vi "Origin_Input.vi"(4 "error in (no error)":errorcluster, 5 "Measured origin x,y":dbl[](array[numeric])=[0.83, 0.79], 6 "Element In":T4, 7 "Outputmode":u16(ring) items=["Get Path", "Make Layout", "Create TRJs"]) -> (0 "error out":errorcluster, 1 "Init Cluster":T7, 2 "TRJs":T5, 3 "Elements Out":T6(array[cluster]))   [LabVIEW 2009]
panel:
  out "output cluster":T1
  in  "Tab Control":enum32{"Main", "Expert", "Output"}(tab)
  in  "Horizontal Line":T2={"Y-Offset"=-9.0, "Length"=9.0, "X-Offset"=25.5}
  in  "Vertical Line":T3={"X-Offset"=20.0, "Length"=7.0, "Y-Offset"=-8.5}
  in  "stop":bool
  in  "Type":i32=4
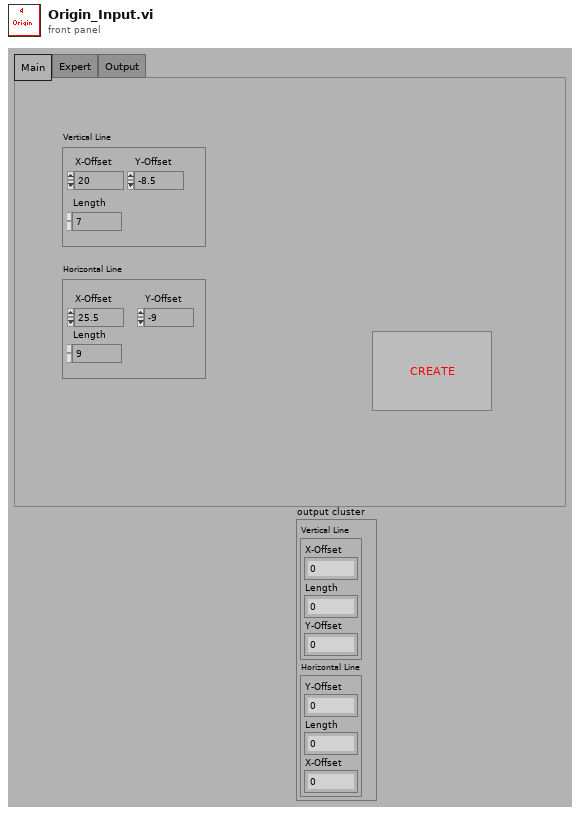
[diagram p1: front panel]
types:
  T1 = cluster{"Vertical Line":cluster{"X-Offset":dbl, "Length":dbl, "Y-Offset":dbl}, "Horizontal Line":cluster{"Y-Offset":dbl, "Length":dbl, "X-Offset":dbl}}
  T2 = cluster{"Y-Offset":dbl, "Length":dbl, "X-Offset":dbl}
  T3 = cluster{"X-Offset":dbl, "Length":dbl, "Y-Offset":dbl}
  T4 = cluster{"Element Name":string, "Type":i32, "Layer per L-Move":i32, "Variant":variant}
  T5 = cluster{"trj file path(1)":path[], "size(s)":i32, dbl[][]}
  T6 = cluster{"Element Name":string, "Type":i32, "Layer per L-Move":i32, "Variant":variant}[]
  T7 = cluster{"path":path, "Button Name":string, "Type":i32}
  T8 = cluster{"Element Name":string, "Value":i32, "Layer per L-Move":i32, "Variant":variant}
  T9 = cluster{"Element Name":string, "Value":i32, "Layer per L-Move":i32, "Variant":variant}[]
  T10 = cluster{"TRJs":path[], i32, "Startpoints":dbl[][]}
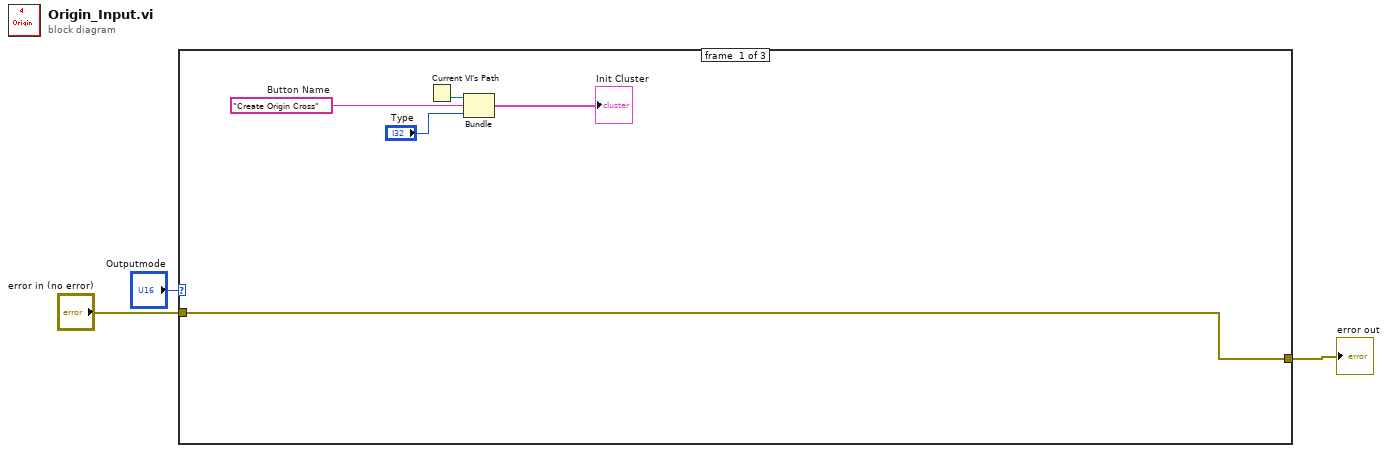
[diagram p0: block diagram]
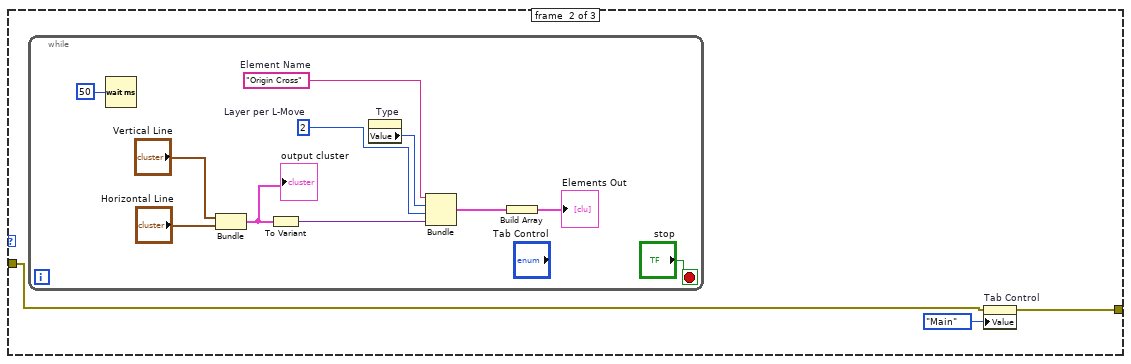
[diagram p2: hidden frame]
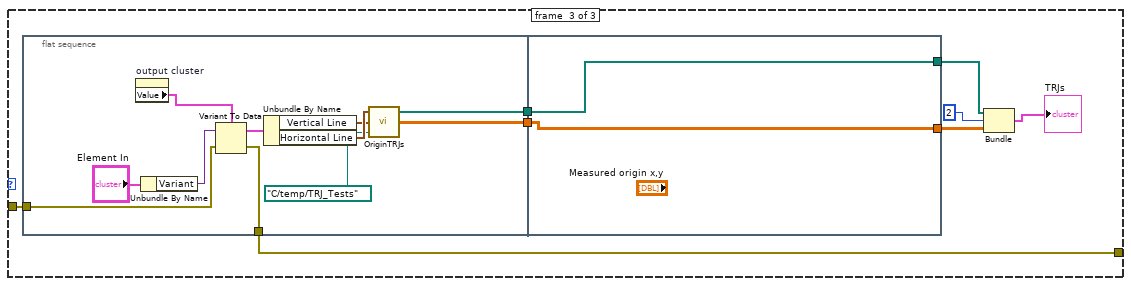
[diagram p3: hidden frame]
diagram:
  n1 = case shown="2" "Outputmode" {
    tunnel: "error in (no error)" -> [w8 w10 w27]
    tunnel: [w8 w9 w26] -> w1
    frame #0 {
      w6 = "Create Origin Cross"  # Button Name
      n2 = Current VI's Path() -> (path=w7:path)
      n3 = Bundle("path"=w7, "Button Name"=w6, "Type"="Type") -> (→"Init Cluster":T7)  [unwired: 1 in]
    }
    frame #1 {
      n4 = while {
        stop <- "stop" stop-if-true
        w17 = 2  # Layer per L-Move
        w20 = "Origin Cross"  # Element Name
        n5 = Wait (ms)(milliseconds to wait=u32 50) -> ()  [unwired: 1 out]
        n6 = Bundle("Vertical Line"="Vertical Line", "Horizontal Line"="Horizontal Line") -> (w14:T1)  [unwired: 1 in]
        "output cluster" <- w14
        n7 = To Variant(anything=w14) -> (Variant=w19:variant)
        n8 = property on="Type" class="DigNum (strict)"() -> ("Value"=w15:i32)  [unwired: 2 in, 2 out]
        n9 = Bundle("Element Name"=w20, "Value"=w15, "Layer per L-Move"=w17, "Variant"=w19) -> (w18:T8)  [unwired: 1 in]
        n10 = Build Array(w18) -> (→"Elements Out":T9)
      }
      n11 = property on="Tab Control" class="TabCtl (strict)"(error in=w10, "Value"=enum32{"Main", "Expert", "Output"}."Main" ("Tab Control")) -> (error out=w9:errorcluster)  [unwired: 1 in, 1 out]
    }
    frame #2 {
      n12 = flat-sequence {
        tunnel: [w37] -> w30
        tunnel: [w36] -> w29
        tunnel: w27 -> [w40]
        tunnel: [w39] -> w26
        tunnel: [w43] -> w28
        tunnel: w30 -> [w43]
        tunnel: w29 -> [w42]
        tunnel: [w42] -> w24
        frame #0 {
          n13 = property on="output cluster" class="Clust (strict)"() -> ("Value"=w32:T1)  [unwired: 2 in, 2 out]
          n14 = Unbundle By Name("Element In") -> ("Variant"=w41:variant)
          n15 = Variant To Data(error in=w40, Variant=w41, type=w32) -> (error out=w39:errorcluster, data=w35:T1)
          n16 = Unbundle By Name(w35) -> ("Vertical Line"=w33:T3, "Horizontal Line"=w34:T2)
          n17 = call "OriginTRJs.vi"("file (use dialog)"=path "C:/temp/TRJ_Tests", "Horizontal Line"=w33, "Vertical Line"=w34) -> ("Startpoints"=w36:dbl[][], "TRJs"=w37:path[])  [unwired: 1 in]
        }
        frame #1 {
        }
      }
      n18 = Bundle("TRJs"=w28, 2, "Startpoints"=w24) -> (→"TRJs":T10)  [unwired: 1 in]
    }
  }
  "error out" <- w1
